vi "Util_Waypoint_To_QuinticInput.vi"(11 "UtilWayPoints":T4[](array[typedef]) {"ANGLE" format="%13.3f"; "Y" format="%13.3f"; "X" format="%13.3f"}) -> (3 "PoseWaypoints":T1[](array[typedef]) {"ROTATION"."SIN" format="%13.4f"; "ROTATION"."COS" format="%13.4f"; "ROTATION"."VALUE" format="%13.4f"; "TRANSLATION"."Y" format="%14.3f"; "TRANSLATION"."X" format="%14.3f"})   [LabVIEW 2019, in "Trajectory_Library.lvlib"]
doc: "Utility function to convert utility waypoints to the input data structures needed to calculate cubic splines."
uses:
  Trajectory_Library.lvlib
  DISPLAY_WAYPOINT.ctl
  TRANSLATION2D.ctl
  ROTATION2D.ctl
  POSE2D.ctl
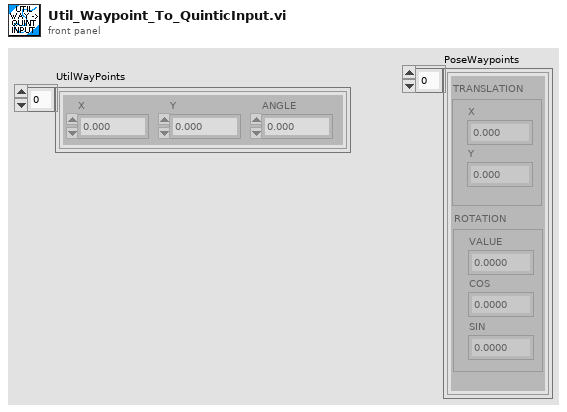
[diagram p1: front panel]
types:
  T1 = typedef "Trajectory_Library.lvlib/POSE2D.ctl" = cluster{"TRANSLATION":T2, "ROTATION":T3}
  T2 = typedef "Trajectory_Library.lvlib/TRANSLATION2D.ctl" = cluster{"X":dbl, "Y":dbl}
  T3 = typedef "Trajectory_Library.lvlib/ROTATION2D.ctl" = cluster{"VALUE":dbl, "COS":dbl, "SIN":dbl}
  T4 = typedef "Trajectory_Library.lvlib/DISPLAY_WAYPOINT.ctl" = cluster{"X":dbl, "Y":dbl, "ANGLE":dbl}
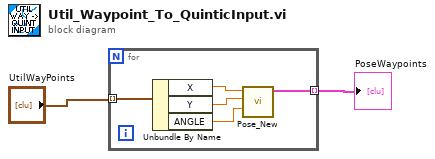
[diagram p0: block diagram]
diagram:
  n1 = for {
    tunnel: "UtilWayPoints" -> [w7] mode=indexing
    tunnel: [w3] -> w1 mode=indexing
    n2 = Unbundle By Name(w7) -> ("X"=w6:dbl, "Y"=w5:dbl, "ANGLE"=w4:dbl)
    n3 = call "Pose_New.vi"("Heading"=w4, "Y"=w5, "X"=w6) -> ("out POSe"=w3:T1)  [unwired: 8 in]
  }
  "PoseWaypoints" <- w1
